vi "Model Initial Values - Export RTM.vi"(8 "error in (no error)":errorcluster, 11 "Node Ptr":u64 format="%.0x") -> (0 "error out":errorcluster)   [LabVIEW 2015, in "Model Initial Values Custom Device.lvlib"]
uses:
  Model Initial Values Custom Device.lvlib
  <vilib>/NI Veristand/Custom Device API/Custom Device API.lvlib
  Model Initial Values - Global.vi
panel:
  # "Please Wait While Export Completes..."
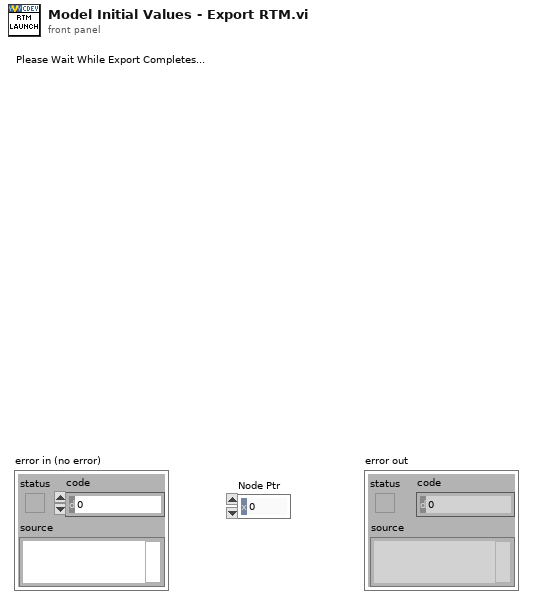
[diagram p1: front panel]
types:
  T1 = cluster{"MultipleSelection":bool, "ShowCheckBox":bool}
  T2 = enum16{"open", "replace", "create", "open or create", "replace or create", "replace or create with confirmation"}
  T3 = typedef "Custom Device API.lvlib/Custom Device Item Info.ctl" = cluster{"Name":string, "Is Channel":bool, "GUID":string, "Is Waveform":bool}
  T4 = typedef "Custom Device API.lvlib/Custom Device Item Ref.ctl" = u64
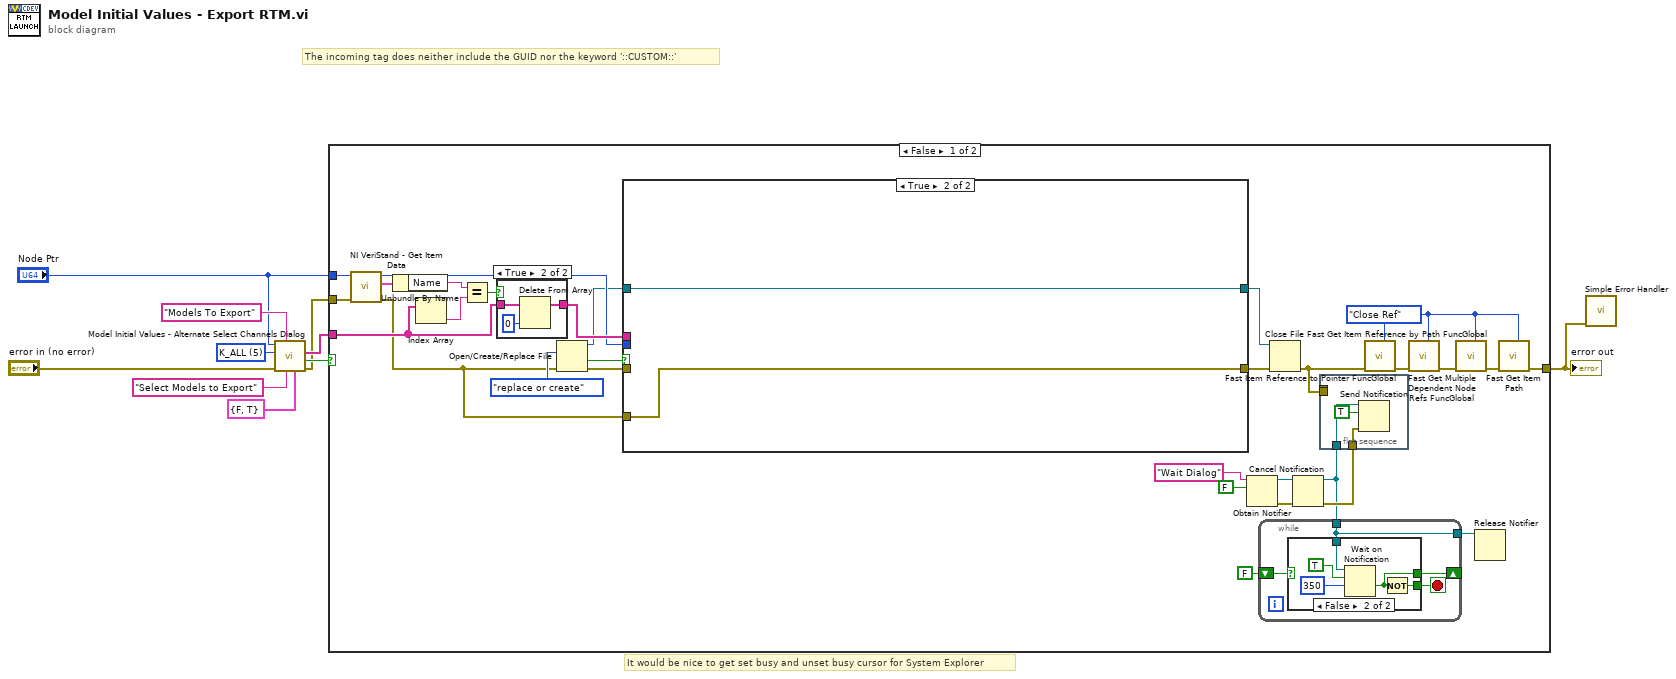
[diagram p0: block diagram]
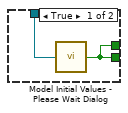
[diagram p2: hidden frame]
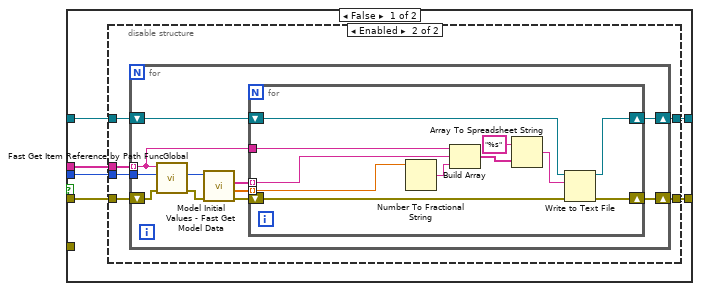
[diagram p3: hidden frame]
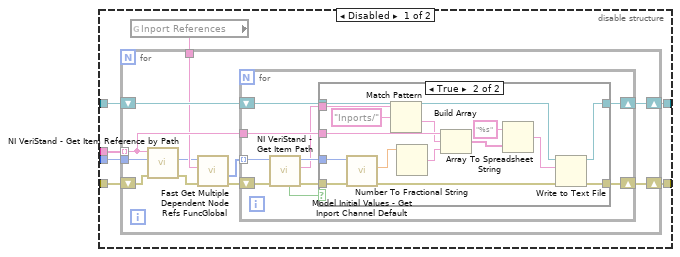
[diagram p4: hidden frame]
diagram:
  w7 = u8 5 items=["K_CHAN_R", "K_CHAN_W", "K_CHAN_RW", "K_CHAN_VOLT", "K_CHAN_FAULT", "K_ALL", "K_CUSTOM"] ("Filter")
  # "It would be nice to get set busy and unset busy cursor for System Explorer"
  # "The incoming tag does neither include the GUID nor the keyword '::CUSTOM::'"
  n1 = call "Model Initial Values - Alternate Select Channels Dialog.vi"("Selection Properties"=T1 {"MultipleSelection"=FALSE, "ShowCheckBox"=TRUE}, "FP Win Title"="Select Models to Export", "Channel Label"="Models To Export", "error in (no error)"="error in (no error)", "Filter"=w7, "Start Item Ref"="Node Ptr") -> ("error out"=w2:errorcluster, "Canceled"=w3:bool, "Channel Names"=w10:string[])  [unwired: 2 in, 1 out]
  n2 = case shown="False" w3 {
    tunnel: w10 -> [w39 _]
    tunnel: w2 -> [w26 w141]
    tunnel: [w13 w141] -> w1
    tunnel: "Node Ptr" -> [w28 _]
    frame False {
      w12 = enum16{"Open or Add", "Close Ref"}."Close Ref" ("Action")
      n3 = call <vilib>:"NI VeriStand - Get Item Data.vi"("error in (no error)"=w26, "Item Ref in"=w28) -> ("error out"=w11:errorcluster, "Item Info"=w34:T3, "Item Ref out"=w35:T4)  [unwired: 6 in, 1 out]
      n4 = Unbundle By Name(w34) -> ("Name"=w36:string)
      n5 = Index Array(array=w39) -> (element=w37:string)  [unwired: 1 in]
      n6 = Equal?(x=w36, y=w37) -> (x = y?=w38:bool)
      n7 = case shown="True" w38 {
        tunnel: w39 -> [w137 w140]
        tunnel: [w137 w138] -> w40
        frame False {
        }
        frame True {
          n8 = Delete From Array(array=w140, index=0) -> (array with subset deleted=w138:string[])  [unwired: 1 in, 1 out]
        }
      }
      n9 = Open/Create/Replace File(error in=w11, operation (0:open)=T2."replace or create") -> (refnum out=w31:refnum<file>, cancelled=w27:bool, error out=w29:errorcluster)  [unwired: 4 in]
      n10 = case shown="True" w27 {
        tunnel: w40 -> [w61 _]
        tunnel: w35 -> [w60 _]
        tunnel: [w59 w136] -> w33
        tunnel: [w56 w135] -> w32
        tunnel: w31 -> [w58 w136]
        tunnel: w29 -> [w57 _]
        tunnel: w11 -> [_ w135]
        frame False {
          n11 = disable-structure shown="Enabled" {
            disable-tunnel: w61 -> [w68 w112]
            disable-tunnel: w60 -> [w67 w111]
            disable-tunnel: [w66 w110] -> w59
            disable-tunnel: w58 -> [w64 w109]
            disable-tunnel: w57 -> [w63 w108]
            disable-tunnel: [w62 w107] -> w56
            frame Disabled {
              n12 = global read "Model Initial Values - Global.vi" "Inport References"() -> (w65:string)
              n13 = for {
                tunnel: w68 -> [w74] mode=indexing
                shift-right: [w79] -> w66
                shift-left: w64 -> [w78]
                shift-right: [w77] -> w62
                shift-left: w63 -> [w75]
                tunnel: w67 -> [w76]
                tunnel: w65 -> [w71]
                n14 = call <vilib>:"NI VeriStand - Get Item Reference by Path.vi"("error in (no error)"=w75, "Root Ref"=w76, "Item Path in"=w74) -> ("error out"=w73:errorcluster, "Item Ref"=w70:T4)  [unwired: 5 in, 2 out]
                n15 = call "Fast Get Multiple Dependent Node Refs FuncGlobal.vi"("error in (no error)"=w73, "Base Property Name"=w71, "Item Ref in"=w70) -> ("error out"=w72:errorcluster, "Dependent Node Refs"=w69:T4[])  [unwired: 6 in, 1 out]
                n16 = for {
                  shift-right: [w89] -> w77
                  shift-left: w72 -> [w84]
                  shift-right: [w87] -> w79
                  shift-left: w78 -> [w88]
                  tunnel: w69 -> [w82] mode=indexing
                  tunnel: w74 -> [w83]
                  n17 = call <vilib>:"NI VeriStand - Get Item Path.vi"("error in (no error)"=w84, "Item Ref in"=w82) -> ("error out"=w86:errorcluster, "Path"=w81:string, "Item Ref out"=w85:T4, "Found"=w80:bool)  [unwired: 6 in]
                  n18 = case shown="True" w80 {
                    tunnel: [w91 w106] -> w89
                    tunnel: w88 -> [w90 w103]
                    tunnel: [w90 w102] -> w87
                    tunnel: w86 -> [w91 w99]
                    tunnel: w85 -> [_ w98]
                    tunnel: w83 -> [_ w95]
                    tunnel: w81 -> [_ w94]
                    frame False {
                    }
                    frame True {
                      n19 = call "Model Initial Values - Get Inport Channel Default.vi"("error in"=w99, "Item Ref in"=w98) -> ("error out"=w97:errorcluster, "Default Value"=w100:dbl)  [unwired: 6 in, 1 out]
                      n20 = Match Pattern(string=w94, regular expression="Inports/") -> (after substring=w93:string)  [unwired: 1 in, 3 out]
                      n21 = Number To Fractional String(number=w100) -> (F-format string=w101:string)  [unwired: 3 in]
                      n22 = Build Array(w95, w93, w101) -> (w96:string[])
                      n23 = Array To Spreadsheet String(array=w96, 3:"%s" ("format string")) -> (spreadsheet string=w104:string)  [unwired: 1 in]
                      n24 = Write to Text File(file (use dialog)=w103, text=w104, error in=w97) -> (refnum out=w102:refnum<file>, error out=w106:errorcluster)  [unwired: 1 in, 1 out]
                    }
                  }
                }
              }
            }
            frame Enabled {
              n25 = for {
                tunnel: w112 -> [w118] mode=indexing
                shift-right: [w123] -> w110
                shift-left: w109 -> [w122]
                shift-right: [w121] -> w107
                shift-left: w108 -> [w119]
                tunnel: w111 -> [w120]
                n26 = call "Fast Get Item Reference by Path FuncGlobal.vi"("error in (no error)"=w119, "Root Ref"=w120, "Item Path in"=w118) -> ("error out"=w116:errorcluster, "Item Ref"=w117:T4)  [unwired: 5 in, 2 out]
                n27 = call "Model Initial Values - Fast Get Model Data.vi"("error in (no error)"=w116, "Local Model Ref in"=w117) -> ("error out"=w115:errorcluster, "Inport Default Values"=w113:dbl[], "Inport Names"=w114:string[])  [unwired: 4 in, 3 out]
                n28 = for {
                  shift-right: [w134] -> w121
                  shift-left: w115 -> [w129]
                  shift-right: [w132] -> w123
                  shift-left: w122 -> [w133]
                  tunnel: w118 -> [w131]
                  tunnel: w114 -> [w124] mode=indexing
                  tunnel: w113 -> [w130] mode=indexing
                  n29 = Number To Fractional String(number=w130) -> (F-format string=w126:string)  [unwired: 3 in]
                  n30 = Build Array(w131, w124, w126) -> (w125:string[])
                  n31 = Array To Spreadsheet String(array=w125, 3:"%s" ("format string")) -> (spreadsheet string=w127:string)  [unwired: 1 in]
                  n32 = Write to Text File(file (use dialog)=w133, text=w127, error in=w129) -> (refnum out=w132:refnum<file>, error out=w134:errorcluster)  [unwired: 1 in, 1 out]
                }
              }
            }
          }
        }
        frame True {
        }
      }
      n33 = Obtain Notifier(name (unnamed)="Wait Dialog", notification data type=FALSE) -> (notifier out=w20:refnum<notifier>, error out=w23:errorcluster)  [unwired: 2 in, 1 out]
      n34 = Close File(refnum=w33, error in=w32) -> (error out=w15:errorcluster)  [unwired: 1 out]
      n35 = Cancel Notification(0:w20, 3:w23) -> (8:w24:refnum<notifier>, 11:w25:errorcluster)  [unwired: 1 out]
      n36 = while {
        tunnel: w24 -> [w41]
        shift-right: [w42] -> _
        shift-left: FALSE -> [w43]
        tunnel: [w41] -> w22
        stop <- w44 stop-if-true
        n37 = case shown="False" w43 {
          tunnel: [w45 w49] -> w44
          tunnel: w41 -> [w46 w51]
          tunnel: [w45 w47] -> w42
          frame True {
            n38 = call "Model Initial Values - Please Wait Dialog.vi"("notifier out"=w46) -> ("Boolean"=w45:bool)
          }
          frame False {
            n39 = Wait on Notification(notifier=w51, ignore previous (F)=TRUE, timeout in ms (-1)=350) -> (timed out?=w47:bool)  [unwired: 1 in, 3 out]
            n40 = Not(x=w47) -> (.not. x?=w49:bool)
          }
        }
      }
      n41 = flat-sequence {
        tunnel: w24 -> [w55]
        tunnel: w25 -> [w54]
        tunnel: [w52] -> _
        tunnel: w15 -> [w52]
        frame #0 {
          n42 = Send Notification(notification=TRUE, notifier=w55, error in (no error)=w54) -> ()  [unwired: 2 out]
        }
      }
      n43 = call "Fast Item Reference to Pointer FuncGlobal.vi"("Action"=w12, "error in (no error)"=w15) -> ("error out"=w16:errorcluster)  [unwired: 6 in, 3 out]
      n44 = call "Fast Get Multiple Dependent Node Refs FuncGlobal.vi"("Action"=w12, "error in (no error)"=w16) -> ("error out"=w17:errorcluster)  [unwired: 7 in, 2 out]
      n45 = call "Fast Get Item Reference by Path FuncGlobal.vi"("Action"=w12, "error in (no error)"=w17) -> ("error out"=w14:errorcluster)  [unwired: 6 in, 3 out]
      n46 = Release Notifier(notifier=w22) -> ()  [unwired: 2 in, 3 out]
      n47 = call "Fast Get Item Path.vi"("Action"=w12, "error in (no error)"=w14) -> ("error out"=w13:errorcluster)  [unwired: 6 in, 3 out]
    }
    frame True {
    }
  }
  "error out" <- w1
  n48 = call <vilib>:"Simple Error Handler.vi"("error in (no error)"=w1) -> ()  [unwired: 4 in, 5 out]
